vi "BRig_Host_dataRunState__entryDelete__delDataPlot__v2.vi"(7 "input_idx":i32[](array[numeric]), 8 "input_col_dataPlot":u16, 9 "input_row_dataPlot":u16, 10 "input_nTrial":u16, 11 "input_dataPlot":u16[][](array[numeric])) -> (0 "output_arrTrials":bool, 3 "output_dataPlot":u16[][](array[numeric]), 4 "output_arrTrials_length":i32, 5 "output_idx":i32[](array[numeric]), 6 "output_arrTrials":i32[](array[numeric]))   [LabVIEW 2014]
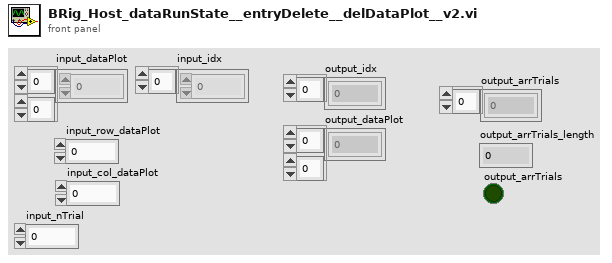
[diagram p1: front panel]
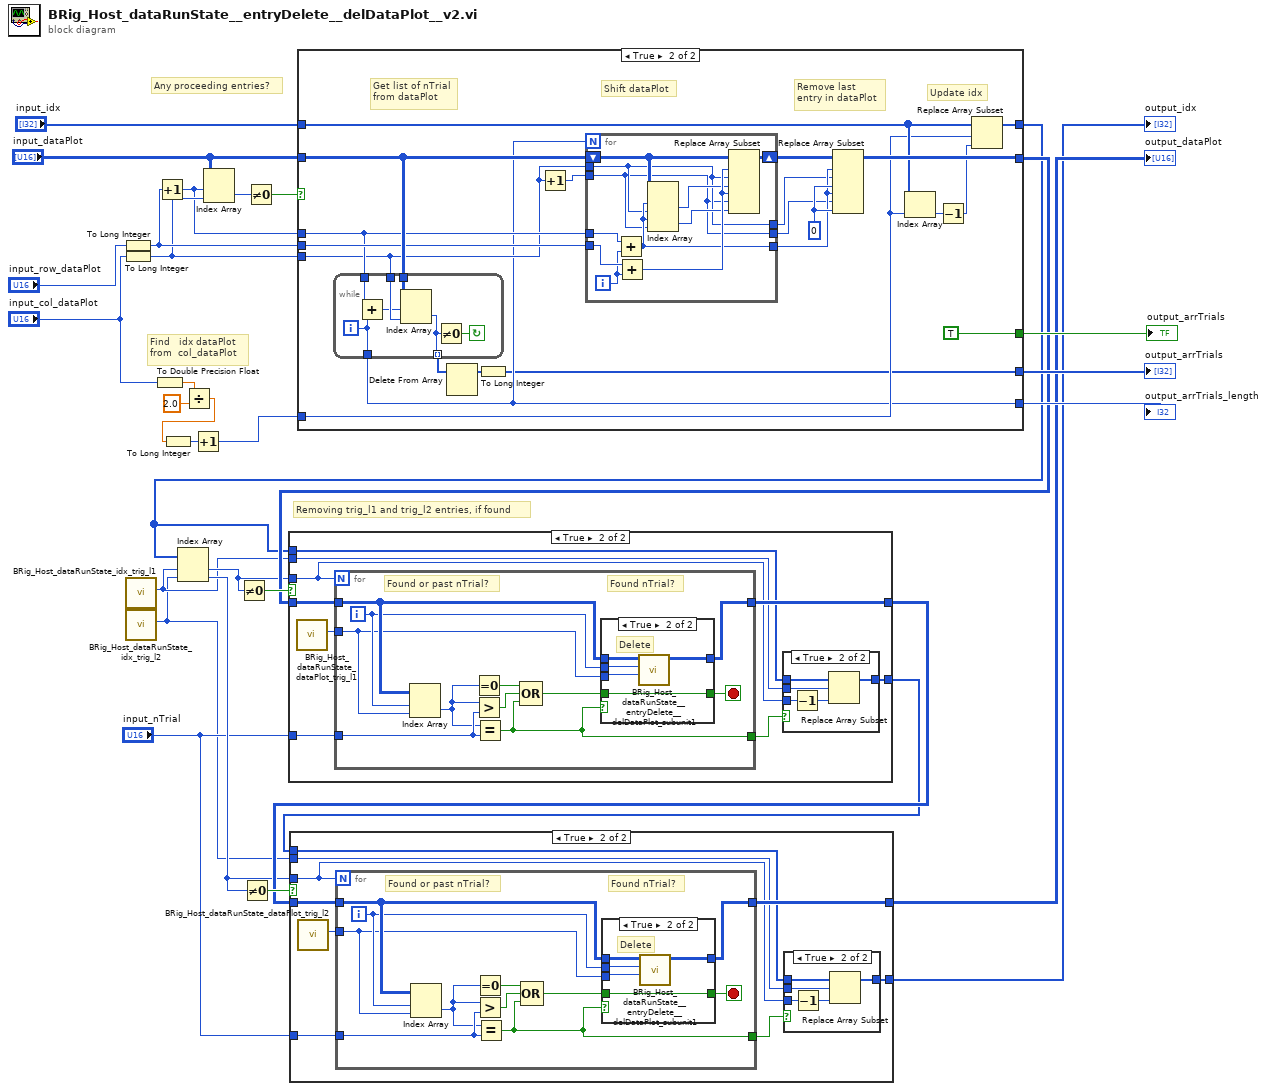
[diagram p0: block diagram]
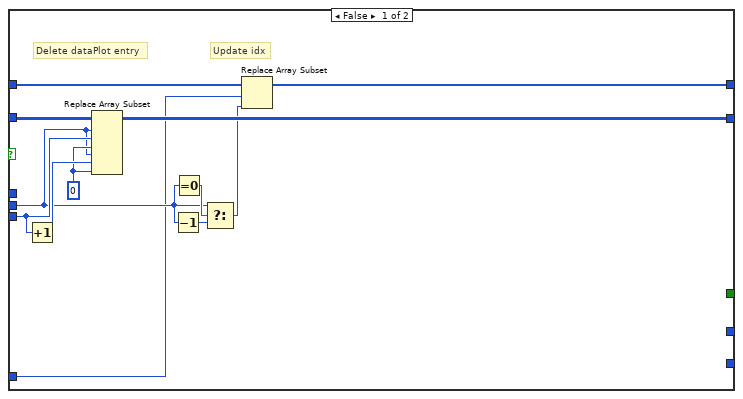
[diagram p8: hidden frame]
diagram:
  # "Removing trig_l1 and trig_l2 entries, if found"
  # "Find   idx dataPlot\nfrom  col_dataPlot"
  # "Any proceeding entries?"
  n1 = To Long Integer(number="input_row_dataPlot") -> (32bit integer=w26:i32)
  n2 = To Long Integer(number="input_col_dataPlot") -> (32bit integer=w25:i32)
  n3 = call "BRig_Host_dataRunState_idx_trig_l1.vi"() -> ("output_idx_trig_l1"=w4:i32)  [unwired: 11 in]
  n4 = call "BRig_Host_dataRunState_idx_trig_l2.vi"() -> ("output_idx_trig_l2"=w3:i32)  [unwired: 11 in]
  n5 = To Double Precision Float(number="input_col_dataPlot") -> (double precision float=w23:dbl)
  n6 = Increment(x=w26) -> (x+1=w24:i32)
  n7 = Divide(x=w23, y=2.0) -> (x/y=w21:dbl)
  n8 = To Long Integer(number=w21) -> (32bit integer=w20:i32)
  n9 = Increment(x=w20) -> (x+1=w18:i32)
  n10 = Index Array(array="input_dataPlot", index (row)=w24, index (col)=w25) -> (element=w29:u16)
  n11 = Not Equal To 0?(x=w29) -> (x != 0?=w28:bool)
  n12 = case shown="True" w28 {
    tunnel: "input_dataPlot" -> [w42 w62]
    tunnel: "input_idx" -> [w37 w50]
    tunnel: w26 -> [w33 w61]
    tunnel: w25 -> [w38 w59]
    tunnel: [w39 w52] -> w13
    tunnel: [w36 w51] -> w10
    tunnel: w24 -> [_ w60]
    tunnel: w18 -> [w31 w47]
    tunnel: [_ w43] -> w17
    tunnel: [_ w46] -> w16
    tunnel: [_ TRUE] -> w15
    frame False {
      w40 = u16 0 ("new element/subarray")
      # "Update idx"
      # "Delete dataPlot entry"
      n13 = Increment(x=w38) -> (x+1=w41:i32)
      n14 = Replace Array Subset(array=w42, new element #1=w40, index (row) #1=w33, index (col) #1=w38, new element #2=w40, index (row) #2=w33, index (col) #2=w41) -> (w39:u16[][])
      n15 = Decrement(x=w33) -> (x-1=w34:i32)
      n16 = Equal To 0?(x=w33) -> (x = 0?=w35:bool)
      n17 = Select(t=w33, s=w35, f=w34) -> (s? t:f=w32:i32)
      n18 = Replace Array Subset(array=w37, new element=w32, index=w31) -> (w36:i32[])
    }
    frame True {
      w57 = u16 0 ("new element/subarray")
      # "Update idx"
      # "Remove last\nentry in dataPlot"
      # "Shift dataPlot"
      # "Get list of nTrial\nfrom dataPlot"
      n19 = while {
        tunnel: w62 -> [w81]
        tunnel: w60 -> [w78]
        tunnel: w59 -> [w80]
        tunnel: [w76] -> w63 mode=indexing
        tunnel: [w75] -> w46
        i -> [w75]
        stop <- w77 continue-if-true
        n20 = Add(x=w78, y=w75) -> (x+y=w79:i32)
        n21 = Index Array(array=w81, index (row)=w79, index (col)=w80) -> (element=w76:u16)
        n22 = Not Equal To 0?(x=w76) -> (x != 0?=w77:bool)
      }
      n23 = Delete From Array(array=w63) -> (array with subset deleted=w44:u16[])  [unwired: 2 in, 1 out]
      n24 = To Long Integer(number=w44) -> (32bit integer=w43:i32[])
      n25 = Increment(x=w59) -> (x+1=w58:i32)
      n26 = for {
        N: w46 -> [_]
        shift-right: [w74] -> w56
        shift-left: w62 -> [w73]
        tunnel: w61 -> [w72]
        tunnel: w60 -> [w70]
        tunnel: w59 -> [w65]
        tunnel: w58 -> [w64]
        tunnel: [w66] -> w55
        tunnel: [w65] -> w54
        tunnel: [w64] -> w53
        i -> [w71]
        n27 = Add(x=w70, y=w71) -> (x+y=w66:i32)
        n28 = Add(x=w72, y=w71) -> (x+y=w69:i32)
        n29 = Index Array(array=w73, index (row) #1=w66, index (col) #1=w65, index (row) #2=w66, index (col) #2=w64) -> (element #1=w68:u16, element #2=w67:u16)
        n30 = Replace Array Subset(array=w73, new element #1=w68, index (row) #1=w69, index (col) #1=w65, new element #2=w67, index (row) #2=w69, index (col) #2=w64) -> (w74:u16[][])
      }
      n31 = Replace Array Subset(array=w56, new element #1=w57, index (row) #1=w55, index (col) #1=w54, new element #2=w57, index (row) #2=w55, index (col) #2=w53) -> (w52:u16[][])
      n32 = Index Array(array=w50, index=w47) -> (element=w49:i32)
      n33 = Decrement(x=w49) -> (x-1=w48:i32)
      n34 = Replace Array Subset(array=w50, new element=w48, index=w47) -> (w51:i32[])
    }
  }
  "output_arrTrials" <- w17
  "output_arrTrials_length" <- w16
  "output_arrTrials" <- w15
  n35 = Index Array(array=w10, index #1=w4, index #2=w3) -> (element #1=w11:i32, element #2=w7:i32)
  n36 = Not Equal To 0?(x=w11) -> (x != 0?=w14:bool)
  n37 = Not Equal To 0?(x=w7) -> (x != 0?=w9:bool)
  n38 = case shown="True" w14 {
    tunnel: w11 -> [_ w86]
    tunnel: w13 -> [w83 w92]
    tunnel: "input_nTrial" -> [_ w90]
    tunnel: [w83 w89] -> w8
    tunnel: w10 -> [w82 w87]
    tunnel: w4 -> [_ w85]
    tunnel: [w82 w84] -> w5
    frame False {
    }
    frame True {
      n39 = call "BRig_Host_dataRunState_dataPlot_trig_l1.vi"() -> ("output_idx_dataPlot_trig_l1"=w91:i32)  [unwired: 11 in]
      n40 = for {
        N: w86 -> [_]
        tunnel: w92 -> [w107]
        tunnel: w91 -> [w105]
        tunnel: w90 -> [w109]
        tunnel: [w103] -> w89
        tunnel: [w102] -> w88
        i -> [w106]
        stop <- w104 stop-if-true
        # "Found nTrial?"
        # "Found or past nTrial?"
        n41 = Index Array(array=w107, index (row)=w106, index (col)=w105) -> (element=w101:u16)
        n42 = Equal To 0?(x=w101) -> (x = 0?=w100:bool)
        n43 = Greater?(x=w101, y=w109) -> (0:w99:bool)
        n44 = Equal?(x=w101, y=w109) -> (x = y?=w102:bool)
        n45 = Compound Arithmetic op=OR(w100, w99, w102) -> (w108:bool)
        n46 = case shown="True" w102 {
          tunnel: w107 -> [w111 w116]
          tunnel: w106 -> [_ w115]
          tunnel: w105 -> [_ w114]
          tunnel: [w111 w113] -> w103
          tunnel: w108 -> [w110 w112]
          tunnel: [w110 w112] -> w104
          frame False {
          }
          frame True {
            # "Delete"
            n47 = call "BRig_Host_dataRunState__entryDelete__delDataPlot_subunit1.vi"("input_col_dataPlot"=w114, "input_row_dataPlot"=w115, "input_dataPlot"=w116) -> ("output_dataPlot"=w113:u16[][])  [unwired: 8 in]
          }
        }
      }
      n48 = case shown="True" w88 {
        tunnel: w87 -> [w93 w97]
        tunnel: w86 -> [_ w98]
        tunnel: w85 -> [_ w96]
        tunnel: [w93 w94] -> w84
        frame False {
        }
        frame True {
          n49 = Decrement(x=w98) -> (x-1=w95:i32)
          n50 = Replace Array Subset(array=w97, new element=w95, index=w96) -> (w94:i32[])
        }
      }
    }
  }
  n51 = case shown="True" w9 {
    tunnel: w7 -> [_ w122]
    tunnel: w8 -> [w118 w127]
    tunnel: "input_nTrial" -> [_ w126]
    tunnel: [w118 w125] -> w2
    tunnel: w5 -> [w117 w123]
    tunnel: w3 -> [_ w121]
    tunnel: [w117 w120] -> w1
    frame False {
    }
    frame True {
      n52 = call "BRig_Host_dataRunState_dataPlot_trig_l2.vi"() -> ("output_idx_dataPlot_trig_l2"=w119:i32)  [unwired: 11 in]
      n53 = for {
        N: w122 -> [_]
        tunnel: w127 -> [w142]
        tunnel: w119 -> [w140]
        tunnel: w126 -> [w144]
        tunnel: [w138] -> w125
        tunnel: [w137] -> w124
        i -> [w141]
        stop <- w139 stop-if-true
        # "Found nTrial?"
        # "Found or past nTrial?"
        n54 = Index Array(array=w142, index (row)=w141, index (col)=w140) -> (element=w136:u16)
        n55 = Equal To 0?(x=w136) -> (x = 0?=w135:bool)
        n56 = Greater?(x=w136, y=w144) -> (0:w134:bool)
        n57 = Equal?(x=w136, y=w144) -> (x = y?=w137:bool)
        n58 = Compound Arithmetic op=OR(w135, w134, w137) -> (w143:bool)
        n59 = case shown="True" w137 {
          tunnel: w142 -> [w146 w151]
          tunnel: w141 -> [_ w150]
          tunnel: w140 -> [_ w149]
          tunnel: [w146 w148] -> w138
          tunnel: w143 -> [w145 w147]
          tunnel: [w145 w147] -> w139
          frame False {
          }
          frame True {
            # "Delete"
            n60 = call "BRig_Host_dataRunState__entryDelete__delDataPlot_subunit1.vi"("input_col_dataPlot"=w149, "input_row_dataPlot"=w150, "input_dataPlot"=w151) -> ("output_dataPlot"=w148:u16[][])  [unwired: 8 in]
          }
        }
      }
      n61 = case shown="True" w124 {
        tunnel: w123 -> [w128 w132]
        tunnel: w122 -> [_ w133]
        tunnel: w121 -> [_ w131]
        tunnel: [w128 w129] -> w120
        frame False {
        }
        frame True {
          n62 = Decrement(x=w133) -> (x-1=w130:i32)
          n63 = Replace Array Subset(array=w132, new element=w130, index=w131) -> (w129:i32[])
        }
      }
    }
  }
  "output_idx" <- w1
  "output_dataPlot" <- w2
